vi "RT Main.vi"() -> ()   [LabVIEW 2014]
uses:
  SubVIs/RT Stop.vi
  <vilib>/Utility/error.llb/Error Cluster From Error Code.vi
  <vilib>/rvi/errors/niLvFpgaAdjustHostInterfaceError.vi
  <vilib>/rvi/interface/nirviReadWriteControl/nirviReadWriteControl.xnode
  NiFpgaLv.dll
  <vilib>/rvi/interface/Simulation/niFpgaSimulationCallBeginRW.vi
panel:
  out "Simulator Timed Out?":bool
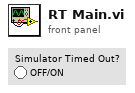
[diagram p1: front panel]
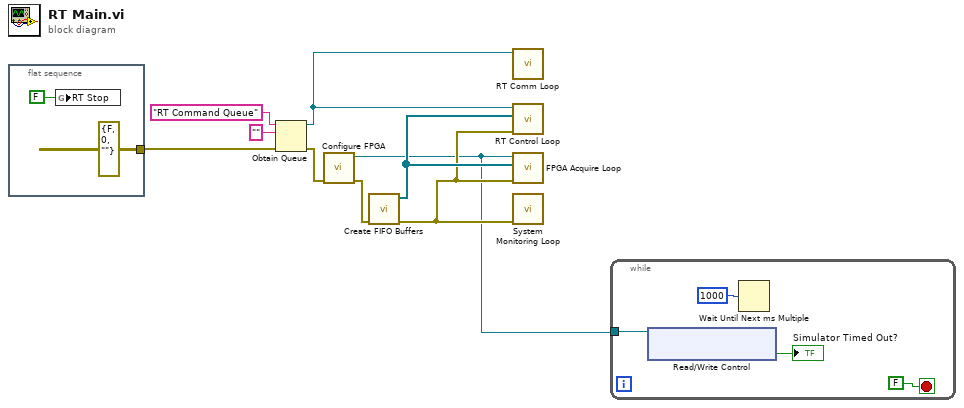
[diagram p0: block diagram]
diagram:
  n1 = flat-sequence {
    tunnel: [errorcluster {"status"=FALSE, "code"=0, "source"=""} ("error in (no error)")] -> w4
    frame #0 {
      n2 = global write "RT Stop.vi" "RT Stop"(FALSE ("RT Stop")) -> ()
    }
  }
  n3 = Obtain Queue(name (unnamed)="RT Command Queue", element data type="", error in (no error)=w4) -> (queue out=w3:refnum<queue>, error out=w8:errorcluster)  [unwired: 2 in, 1 out]
  n4 = call "Configure FPGA.vi"("error in"=w8) -> ("error out"=w6:errorcluster, "Refnum out"=w1:refnum<k20>)  [unwired: 9 in]
  n5 = call "Create FIFO Buffers.vi"("error in (no error)"=w6) -> ("error out"=w2:errorcluster, "FIFO Buffers"=w5:refnum<k33>[])  [unwired: 9 in]
  n6 = call "RT Comm Loop.vi"("Queue in"=w3) -> ()  [unwired: 11 in]
  n7 = call "RT Control Loop.vi"("error in (no error)"=w2, "FIFO Buffers"=w5, "Queue in"=w3) -> ()  [unwired: 9 in]
  n8 = call "FPGA Acquire Loop.vi"("error in (no error)"=w2, "FIFO Buffers"=w5, "Refnum in"=w1) -> ()  [unwired: 9 in]
  n9 = call "System Monitoring Loop.vi"("error in (no error)"=w2) -> ()  [unwired: 11 in]
  n10 = while {
    tunnel: w1 -> [w15]
    stop <- FALSE stop-if-true
    n11 = xnode "Read/Write Control"("FPGA VI Reference In"=w15) -> ("Simulator Timed Out?"=→"Simulator Timed Out?":bool)  [unwired: 1 in, 2 out]
    n12 = Wait Until Next ms Multiple(millisecond multiple=u32 1000) -> ()  [unwired: 1 out]
  }
